vi "Build Picture.vi"(9 "Energized Picture":T1, 10 "Feedback Picture":T1, 11 "Command Picture":T1) -> (2 "Valve Picture":picture)   [LabVIEW 2020, in "VolatusGUI.lvlib" / "2WayValve.lvclass"]
uses:
  2WayValve.lvclass
  Picture.ctl
  2WayValve.lvclass/2WayValve.ctl
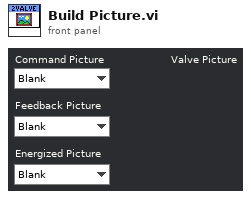
[diagram p1: front panel]
types:
  T1 = typedef "VolatusGUI.lvlib/2WayValve.lvclass/Picture.ctl" = enum16{"Blank", "OuterV", "OuterH", "OuterI", "OuterC", "OuterS", "OuterE", "InnerV", "InnerH", "InnerI", "InnerC", "InnerS", "InnerE", "EnergizedDe", "EnergizedEn", "EnergizedC", "EnergizedS", "EnergizedEr"}
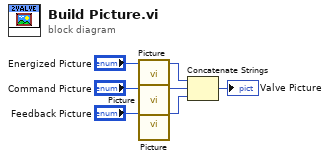
[diagram p0: block diagram]
diagram:
  n1 = call "Picture.vi"("Picture Item"="Energized Picture") -> ("Picture"=w1:picture)  [unwired: 10 in]
  n2 = call "Picture.vi"("Picture Item"="Command Picture") -> ("Picture"=w4:picture)  [unwired: 10 in]
  n3 = call "Picture.vi"("Picture Item"="Feedback Picture") -> ("Picture"=w3:picture)  [unwired: 10 in]
  n4 = Concatenate Strings(w1, w4, w3) -> (→"Valve Picture":picture)
